vi "Decimal to ascii converstion.vi"(10 "DECIMAL VALUE":u16[](array[numeric])) -> (2 "array w/ subset deleted":string[](array[string]))   [LabVIEW 2017]
panel:
  out "trimmed string":string
  out "BARCODE":string
  out "ASCII VALUE":string[](array[string])
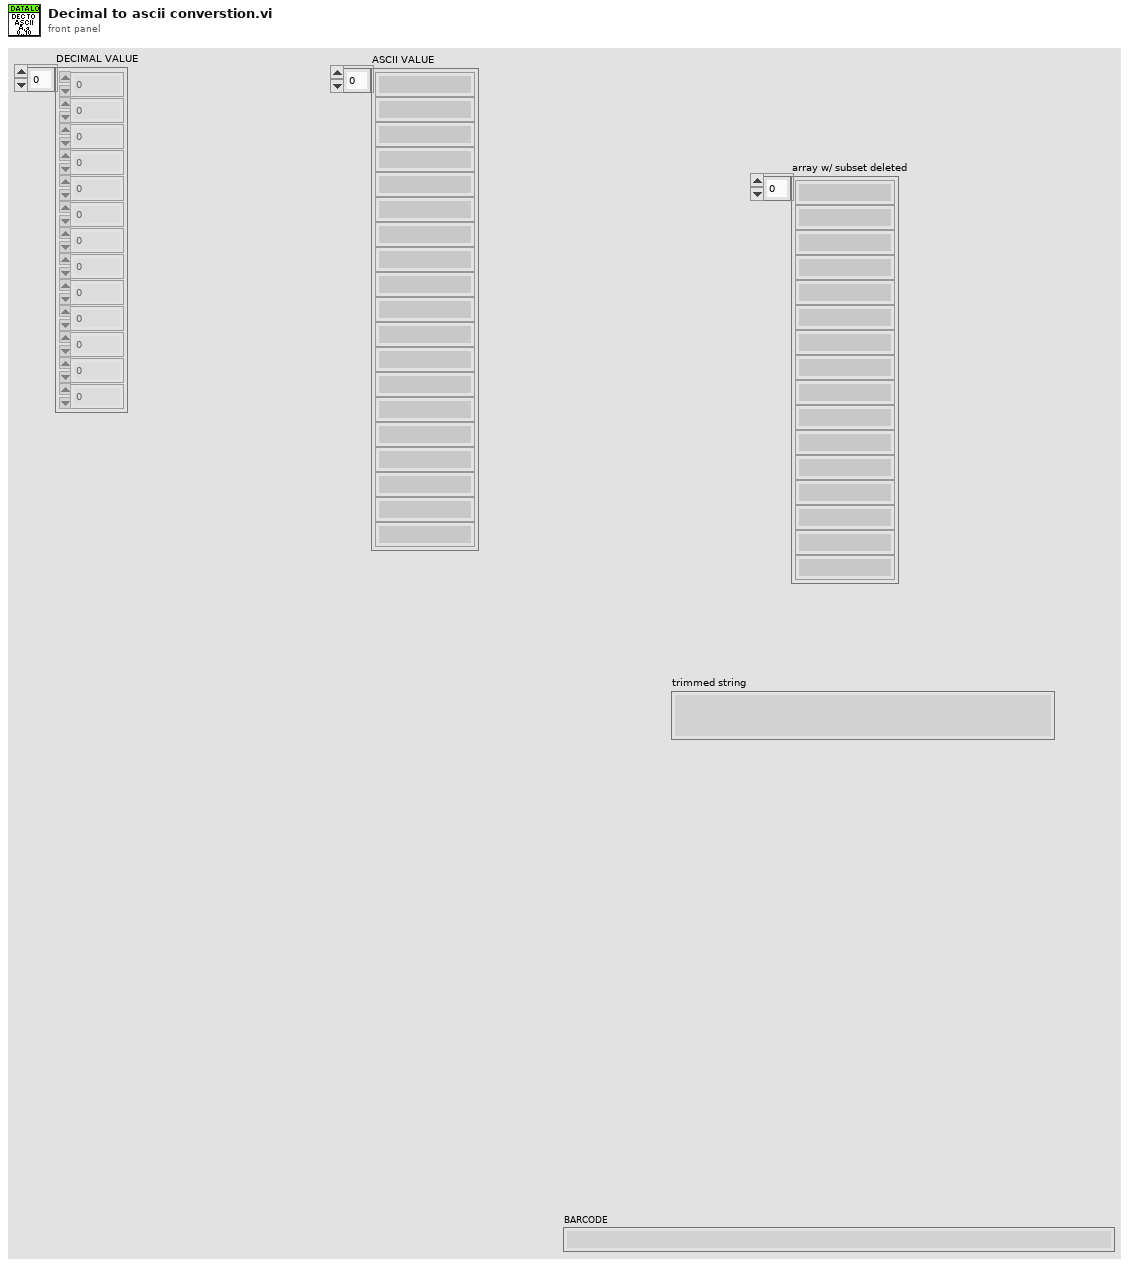
[diagram p1: front panel]
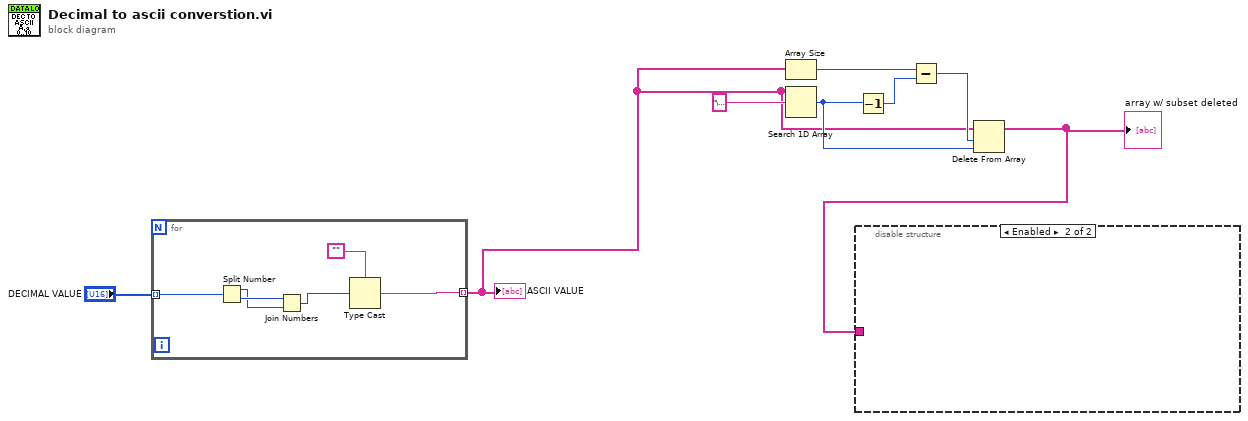
[diagram p0: block diagram]
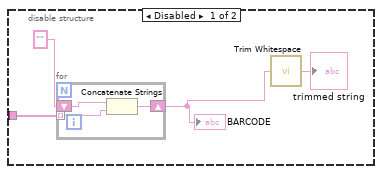
[diagram p2: hidden frame]
diagram:
  n1 = for {
    tunnel: [w9] -> w2 mode=indexing
    tunnel: "DECIMAL VALUE" -> [w11] mode=indexing
    n2 = Split Number(x=w11) -> (hi(x)=w12:u8, lo(x)=w13:u8)
    n3 = Join Numbers(hi=w13, lo=w12) -> ((hi.lo)=w10:u16)
    n4 = Type Cast(type="", x=w10) -> (*(type *) &x=w9:string)
  }
  "ASCII VALUE" <- w2
  n5 = Array Size(array=w2) -> (size(s)=w3:i32)
  n6 = Search 1D Array(1D array=w2, element="\u0000\u0000") -> (index of element=w6:i32)  [unwired: 1 in]
  n7 = Decrement(x=w6) -> (x-1=w5:i32)
  n8 = Subtract(x=w3, y=w5) -> (x-y=w4:i32)
  n9 = Delete From Array(array=w2, length=w4, index=w6) -> (array with subset deleted=w1:string[])  [unwired: 1 out]
  "array w/ subset deleted" <- w1
  n10 = disable-structure shown="Enabled" {
    disable-tunnel: w1 -> [w15 _]
    frame Disabled {
      n11 = for {
        tunnel: w15 -> [w21] mode=indexing
        shift-right: [w20] -> w17
        shift-left: "" -> [w19]
        n12 = Concatenate Strings(w19, w21) -> (w20:string)
      }
      "BARCODE" <- w17
      n13 = call <vilib>:"Trim Whitespace.vi"("string"=w17) -> ("trimmed string"=→"trimmed string":string)  [unwired: 1 in]
    }
    frame Enabled {
    }
  }
